vi "tesla2kA.vi"(2 "Magnet Filed [T]":dbl=1.0 format="%.4f") -> (0 "Current [kA]":dbl=1.0 format="%.4f")   [LabVIEW 2019]
uses:
  PS Comm Globals.vi
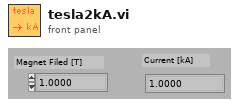
[diagram p1: front panel]
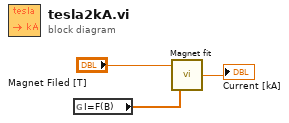
[diagram p0: block diagram]
diagram:
  n1 = global read "PS Comm Globals.vi" "I=F(B)"() -> (w2:dbl[])
  n2 = call "Magnet fit.vi"("Coefficients"=w2, "Magnet Parameter"="Magnet Filed [T]") -> ("Conjugate Parameter"=→"Current [kA]":dbl)
